vi "Slide Stitching.vi"() -> ()   [LabVIEW 2017]
uses:
  <vilib>/vision/Image Controls.llb/IMAQ Image.ctl
  <vilib>/vision/NI_Vision_Development_Module.lvlib
panel:
  out "error out":errorcluster
  out "Y Resolution 2":i32
  out "X Resolution 3":i32
  out "Final Stiched Image":T1(plugin-control)
  out "Image Out 3":T1
  out "Array 8":i32[](array[numeric])
  out "Array 7":i32[](array[numeric])
  out "Number of Files":i32
  out "Images 2":T1[](array[plugin-control])
  out "Stiched Image 2":T1(plugin-control)
  out "X Resolution 2":i32
  out "Image Out 2":T1
  out "Array 5":i32[](array[numeric])
  out "Array 4":T1[](array[plugin-control])
  out "Array 3":T1[](array[plugin-control])
  out "Array 2":i32[](array[numeric])
  out "Image Out":T1
  out "X Resolution":i32
  out "Y Resolution":i32
  out "Array":i32[](array[numeric])
  out "Image Type":T2 items=["Grayscale (U8)", "Grayscale (I16)", "Grayscale (SGL)", "Complex (CSG)", "RGB (U32)", "HSL (U32)", "RGB (U64)", "Grayscale (U16)"]
  out "Images":T1[](array[plugin-control])
  out "Stiched Image 1":T1(plugin-control)
  # "Overview: Demonstrates how to stitch multiple images into a big image.\nRequirements: LabVIEW Base Development System 2012 (or compatible)\n                             NI Vision Development Module 2012 (or compatible)\nInstructions: \n1. Run the VI."
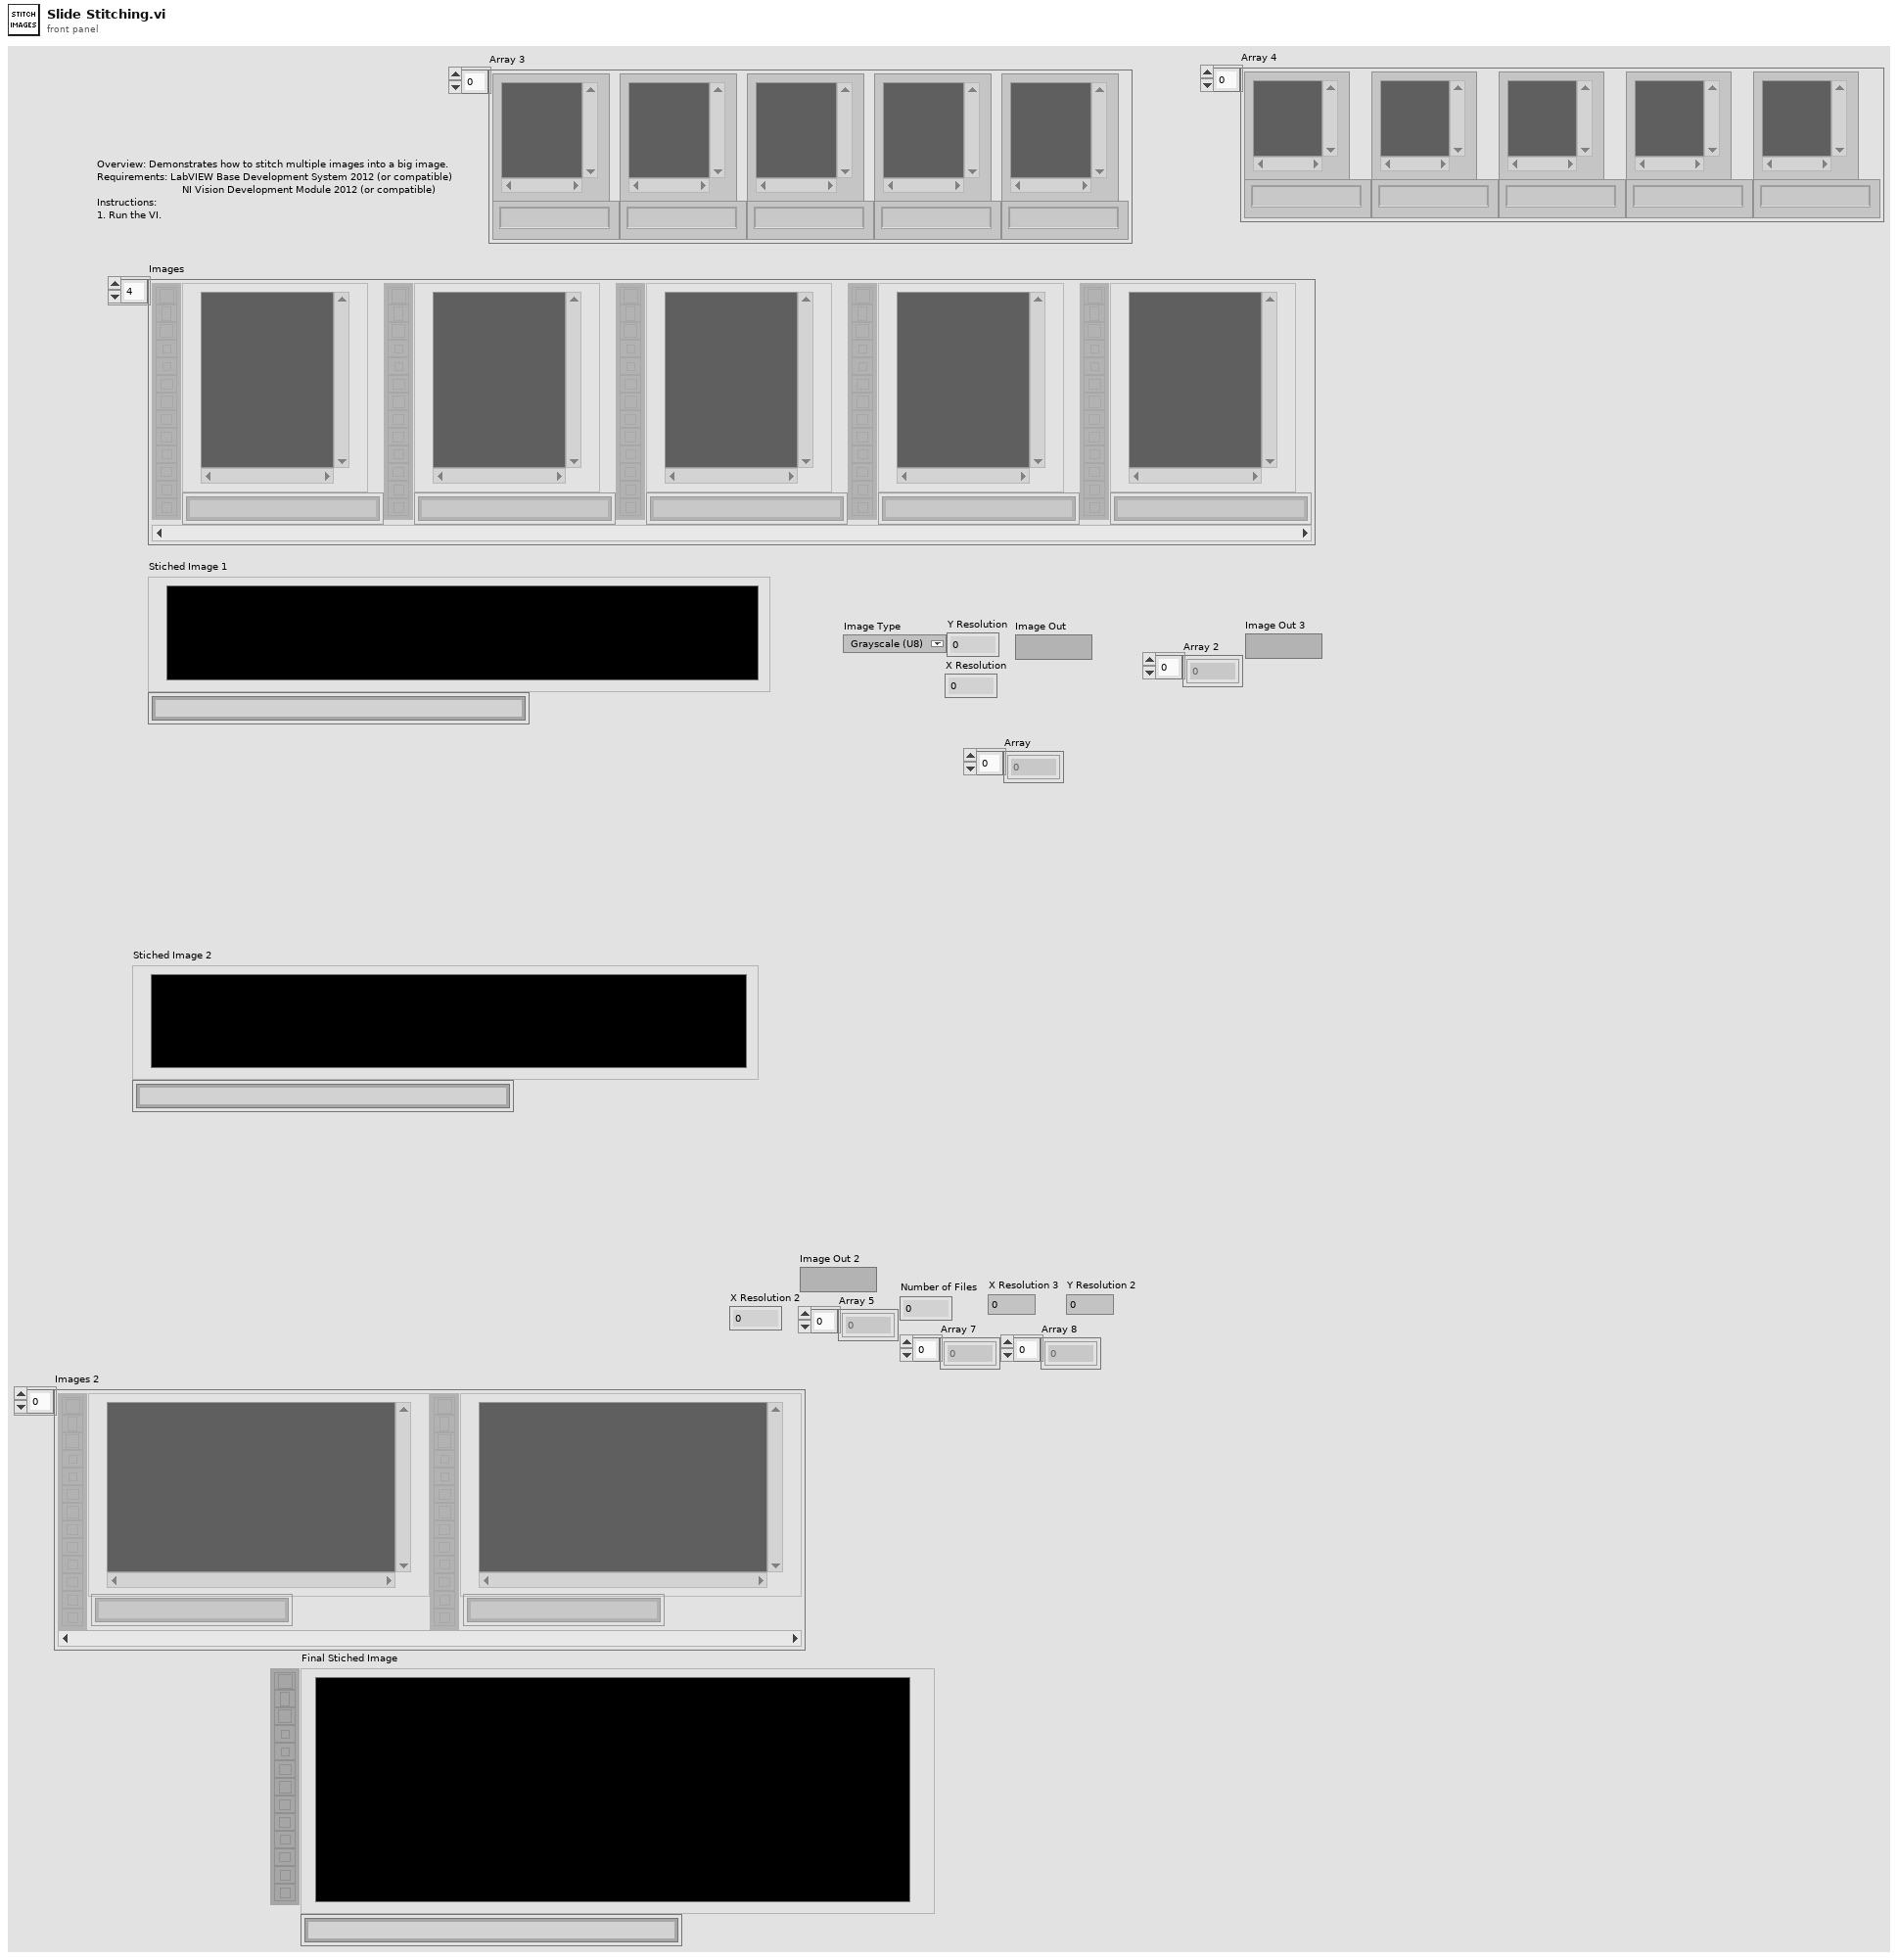
[diagram p1: front panel]
types:
  T1 = typedef "IMAQ Image.ctl" = refnum<image>
  T2 = typedef "Image Type" = u32
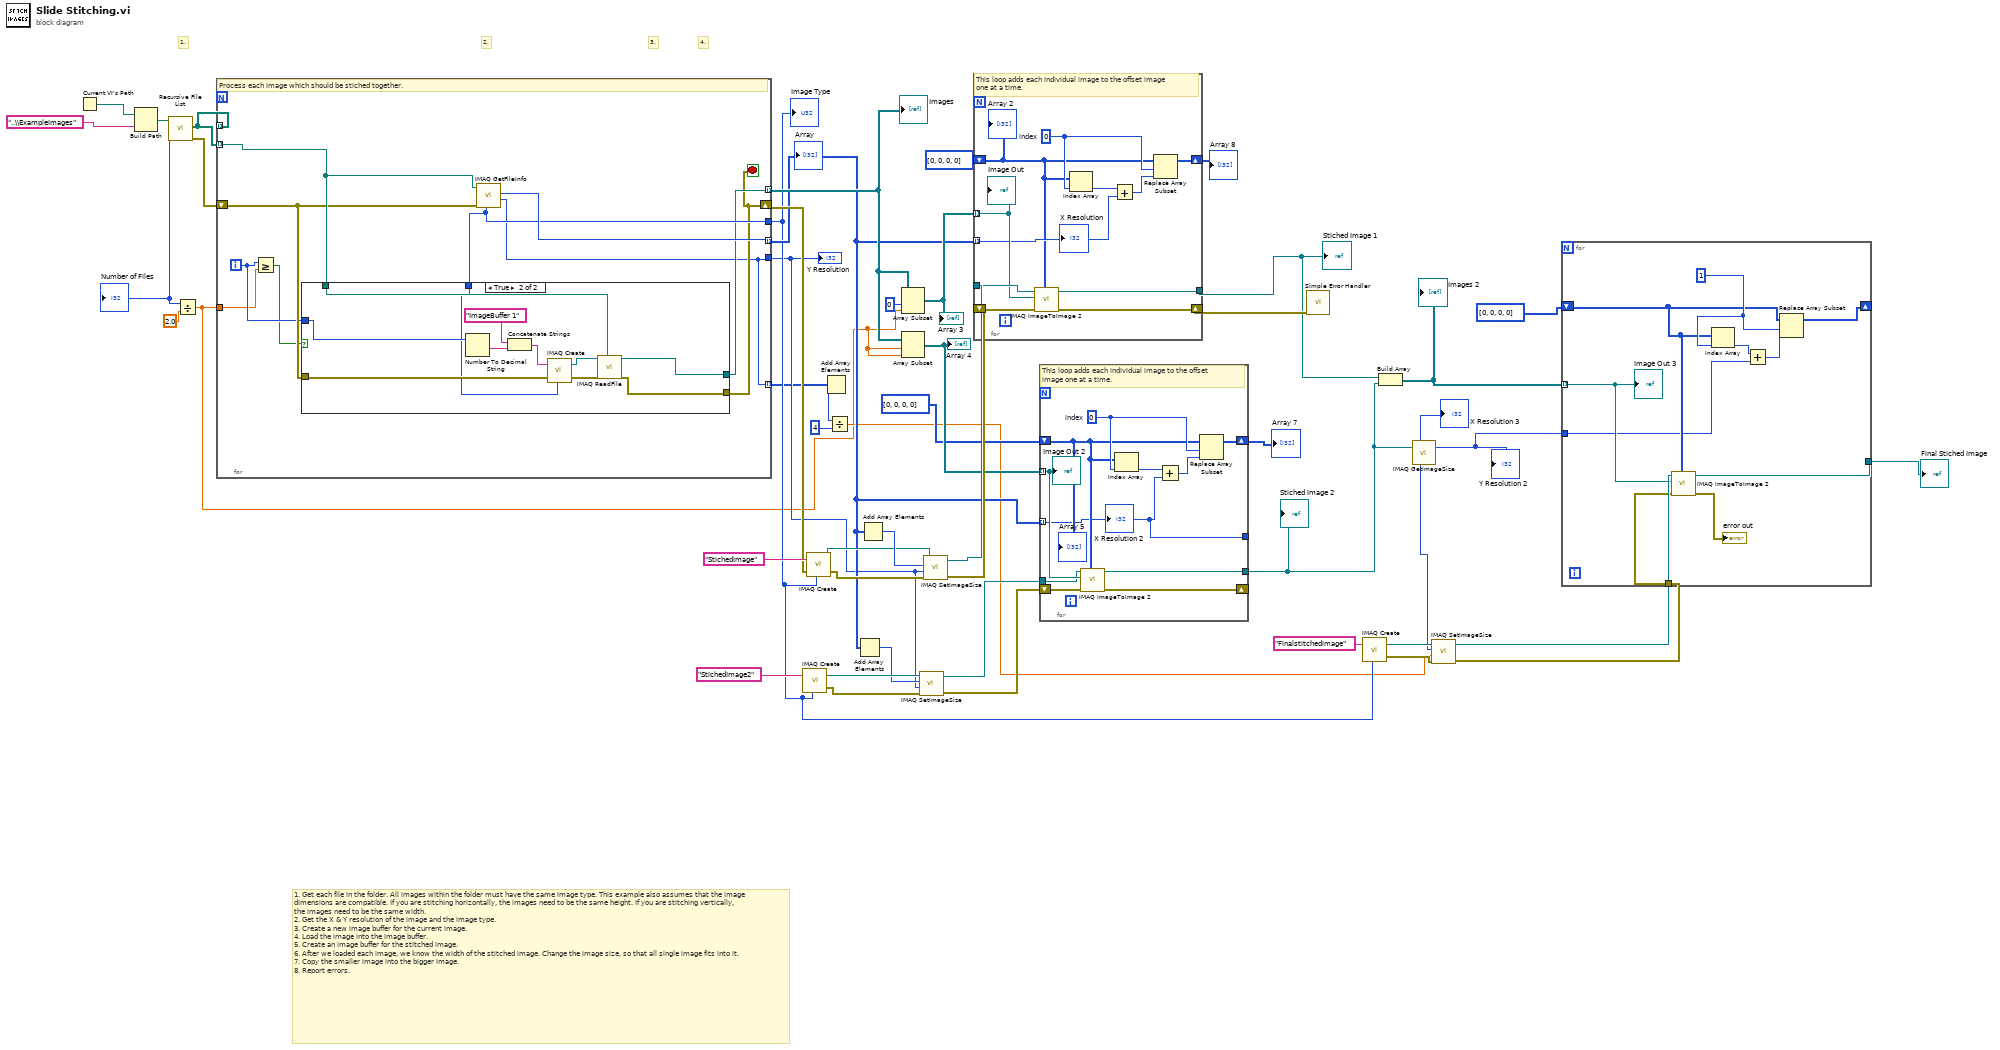
[diagram p0: block diagram]
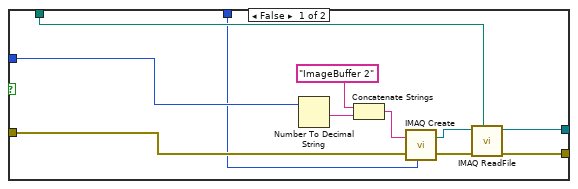
[diagram p2: hidden frame]
diagram:
  # "1. Get each file in the folder. All images within the folder must have the same image type. This example also assumes that the image dimensions are compatible. If you are stitching horizontally, the images need to be the same height. If you are stitching vertically, the images need to be the same width.\n2. Get the X & Y resolution of the image and the image type.\n3. Create a new image buffer for the current image.\n4. Load the image into the image buffer.\n5. Create an image buffer for the stitched image.\n6. After we loaded each image, we know the width of the stitched image. Change the image size, so that all single image fits into it.\n7. Copy the smaller image into the bigger image.\n8. Report errors."
  # "4."
  # "3."
  # "2."
  # "1."
  n1 = Current VI's Path() -> (path=w47:path)
  n2 = Build Path(base path=w47, name or relative path="..\\ExampleImages") -> (appended path=w46:path)
  n3 = call <vilib>:"Recursive File List.vi"("Folder Path"=w46) -> ("error out"=w39:errorcluster, "Number of Files"=w2:i32, "All Files in Dir"=w36:path[])  [unwired: 6 in, 2 out]
  "Number of Files" <- w2
  n4 = Divide(x=w2, y=2.0) -> (x/y=w1:dbl)
  n5 = for {
    tunnel: [w53] -> w35 mode=indexing
    shift-right: [w52] -> w38
    shift-left: w39 -> [w57]
    tunnel: w36 -> [_] mode=indexing
    tunnel: [w59] -> w25 mode=indexing
    tunnel: [w51] -> w15
    tunnel: [w54] -> w18
    tunnel: w36 -> [w58] mode=indexing
    tunnel: [w51] -> w8 mode=indexing
    tunnel: w1 -> [w50]
    i -> [w56]
    stop <- w52 stop-if-true
    # "Process each image which should be stiched together."
    n6 = Greater Or Equal?(x=w56, y=w50) -> (x >= y?=w55:bool)
    n7 = call "IMAQ GetFileInfo"("error in (no error)"=w57, "File Path"=w58) -> ("Y Resolution"=w51:i32, "X Resolution"=w59:i32, "Image Type"=w54:T2)  [unwired: 3 in, 4 out]
    n8 = case shown="True" w55 {
      tunnel: w58 -> [w63 w76]
      tunnel: w57 -> [w64 w75]
      tunnel: w56 -> [w65 w74]
      tunnel: w54 -> [w62 w73]
      tunnel: [w61 w72] -> w52
      tunnel: [w60 w71] -> w53
      frame False {
        n9 = Number To Decimal String(number=w65) -> (decimal integer string=w66:string)  [unwired: 1 out]
        n10 = Concatenate Strings("ImageBuffer 2", w66) -> (w70:string)
        n11 = call "IMAQ Create"("Image Name"=w70, "Image Type"=w62, "error in (no error)"=w64) -> ("New Image"=w69:T1, "error out"=w68:errorcluster)  [unwired: 1 in, 1 out]
        n12 = call "IMAQ ReadFile"("File Path"=w63, "error in (no error)"=w68, "Image"=w69) -> ("error out"=w61:errorcluster, "Image Out"=w60:T1)  [unwired: 2 in, 5 out]
      }
      frame True {
        n13 = Number To Decimal String(number=w74) -> (decimal integer string=w77:string)  [unwired: 1 out]
        n14 = Concatenate Strings("ImageBuffer 1", w77) -> (w81:string)
        n15 = call "IMAQ Create"("Image Name"=w81, "Image Type"=w73, "error in (no error)"=w75) -> ("New Image"=w80:T1, "error out"=w79:errorcluster)  [unwired: 1 in, 1 out]
        n16 = call "IMAQ ReadFile"("File Path"=w76, "error in (no error)"=w79, "Image"=w80) -> ("error out"=w72:errorcluster, "Image Out"=w71:T1)  [unwired: 2 in, 5 out]
      }
    }
  }
  "Images" <- w35
  "Image Type" <- w18
  "Array" <- w25
  "Y Resolution" <- w15
  n17 = call "IMAQ Create"("Image Name"="StichedImage2", "Image Type"=w18) -> ("New Image"=w32:T1, "error out"=w33:errorcluster)  [unwired: 2 in, 1 out]
  n18 = call "IMAQ Create"("Image Name"="StichedImage", "Image Type"=w18, "error in (no error)"=w38) -> ("New Image"=w44:T1, "error out"=w37:errorcluster)  [unwired: 1 in, 1 out]
  n19 = Add Array Elements(numeric array=w8) -> (sum=w6:i32)
  n20 = Divide(x=w6, y=4) -> (x/y=w5:dbl)
  n21 = Add Array Elements(numeric array=w25) -> (sum=w31:i32)
  n22 = Add Array Elements(numeric array=w25) -> (sum=w45:i32)
  n23 = Array Subset(array=w35, index=0, length=w1) -> (w29:T1[])
  "Array 3" <- w29
  n24 = Array Subset(array=w35, index=w1, length=w1) -> (w28:T1[])
  "Array 4" <- w28
  n25 = call "IMAQ SetImageSize"("error in (no error)"=w33, "Y Resolution"=w15, "X Resolution"=w31, "Image"=w32) -> ("error out"=w26:errorcluster, "Image Out"=w27:T1)  [unwired: 1 out]
  n26 = call "IMAQ SetImageSize"("error in (no error)"=w37, "Y Resolution"=w15, "X Resolution"=w45, "Image"=w44) -> ("error out"=w42:errorcluster, "Image Out"=w43:T1)  [unwired: 1 out]
  n27 = for {
    tunnel: w43 -> [w92]
    tunnel: w29 -> [w91] mode=indexing
    shift-right: [w89] -> w40
    shift-left: w42 -> [w90]
    tunnel: [w88] -> w23
    shift-right: [w87] -> w21
    shift-left: i32[] [0, 0, 0, 0] -> [w82]
    tunnel: w25 -> [w83] mode=indexing
    w86 = 0  # index
    # "This loop adds each individual image to the offset image one at a time."
    n28 = call "IMAQ ImageToImage 2"("Offset Left/Top"=w82, "error in (no error)"=w90, "Image Src (Small)"=w91, "Image Src (Large)"=w92) -> ("error out"=w89:errorcluster, "Image Dst Out"=w88:T1)  [unwired: 2 in, 4 out]
    n29 = Index Array(array=w82, index=w86) -> (element=w84:i32)
    n30 = Add(x=w84, y=w83) -> (x+y=w85:i32)
    n31 = Replace Array Subset(array=w82, new element=w85, index=w86) -> (w87:i32[])
    "X Resolution" <- w83
    "Image Out" <- w91
    "Array 2" <- w82
  }
  "Stiched Image 1" <- w23
  "Array 8" <- w21
  n32 = for {
    tunnel: w28 -> [w103] mode=indexing
    shift-right: [w101] -> _
    shift-left: w26 -> [w102]
    tunnel: [w100] -> w12
    shift-right: [w99] -> w22
    shift-left: i32[] [0, 0, 0, 0] -> [w95]
    tunnel: w25 -> [w93] mode=indexing
    tunnel: w27 -> [w94]
    tunnel: [w93] -> _
    w98 = 0  # index
    # "This loop adds each individual image to the offset image one at a time."
    n33 = call "IMAQ ImageToImage 2"("Offset Left/Top"=w95, "error in (no error)"=w102, "Image Src (Small)"=w103, "Image Src (Large)"=w94) -> ("error out"=w101:errorcluster, "Image Dst Out"=w100:T1)  [unwired: 2 in, 4 out]
    n34 = Index Array(array=w95, index=w98) -> (element=w96:i32)
    n35 = Add(x=w96, y=w93) -> (x+y=w97:i32)
    n36 = Replace Array Subset(array=w95, new element=w97, index=w98) -> (w99:i32[])
    "X Resolution 2" <- w93
    "Image Out 2" <- w103
    "Array 5" <- w95
  }
  "Stiched Image 2" <- w12
  "Array 7" <- w22
  n37 = call <vilib>:"Simple Error Handler.vi"("error in (no error)"=w40) -> ()  [unwired: 4 in, 5 out]
  n38 = call "IMAQ Create"("Image Name"="Finalstitchedimage", "Image Type"=w18) -> ("New Image"=w16:T1, "error out"=w17:errorcluster)  [unwired: 2 in, 1 out]
  n39 = Build Array(w23, w12) -> (w13:T1[])
  "Images 2" <- w13
  n40 = call "IMAQ GetImageSize"("Image"=w12) -> ("Y Resolution"=w4:i32, "X Resolution"=w11:i32)  [unwired: 3 in, 1 out]
  "X Resolution 3" <- w11
  "Y Resolution 2" <- w4
  n41 = call "IMAQ SetImageSize"("error in (no error)"=w17, "Y Resolution"=w5, "X Resolution"=w11, "Image"=w16) -> ("error out"=w9:errorcluster, "Image Out"=w14:T1)  [unwired: 1 out]
  n42 = for {
    tunnel: w13 -> [w108] mode=indexing
    shift-right: [w112] -> _
    shift-left: i32[] [0, 0, 0, 0] -> [w110]
    tunnel: w14 -> [w109]
    tunnel: [w107] -> w10
    tunnel: w9 -> [w106]
    tunnel: w4 -> [w105]
    w111 = 1 ("index")
    n43 = call "IMAQ ImageToImage 2"("Offset Left/Top"=w110, "error in (no error)"=w106, "Image Src (Small)"=w108, "Image Src (Large)"=w109) -> ("error out"=→"error out":errorcluster, "Image Dst Out"=w107:T1)  [unwired: 2 in, 4 out]
    n44 = Index Array(array=w110, index=w111) -> (element=w114:i32)
    n45 = Add(x=w114, y=w105) -> (x+y=w113:i32)
    n46 = Replace Array Subset(array=w110, new element=w113, index=w111) -> (w112:i32[])
    "Image Out 3" <- w108
  }
  "Final Stiched Image" <- w10
